vi "Using Connection Strings.vi"() -> ()   [LabVIEW 2012]
doc: "This example shows how to build an executable that uses the Database Connectivity Toolkit. It also shows how to dynamically create a connection string so the database being used can move with the executable."
uses:
  NI_Database_API_64.lvlib
  _DB Variant To Data/Database Variant To Data.xnode
  Connection.llb/DB Tools Open Connec (String).vi
  Auxilliary.llb/DB Tools Cursor Type.ctl
  Connection.llb/Conn Execute.vi
  Recordset.llb/Rec Get Recordset Properties (R).vi
  Recordset.llb/Rec Move To Record N (R).vi
  Recordset.llb/Rec Fetch Recordset Data (R).vi
  Recordset.llb/Rec Destroy - Connection.vi
panel:
  out "String read from database":string
  out "Numeric read from database":i32
  out "Date/Time read from database":timestamp format="%<%X\n%x>T"
  in  "String to insert":string="this is a test."
  in  "Numeric to insert":i32=125
  out "Date/Time inserted":timestamp format="%<%X\n%x>T"
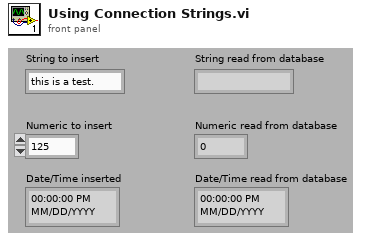
[diagram p1: front panel]
types:
  T1 = typedef "NI_Database_API_64.lvlib/DB Tools Cursor Type.ctl" = enum16{"forward-only", "keyset", "dynamic", "static"}
  T2 = enum32{"invalid app kind", "Development System", "Run Time System", "Student Edition", "Embedded LabVIEW", "Evaluation", "Custom"}
  T3 = typedef "NI_Database_API_64.lvlib/Conn ObjectReference.ctl" = refnum<k1>
  T4 = cluster{"String to insert":string, "Numeric to insert":i32, "seconds since 1Jan1904":timestamp}
  T5 = typedef "NI_Database_API_64.lvlib/Rec ObjectReference.ctl" = refnum<k1>
  T6 = typedef "NI_Database_API_64.lvlib/Rec Properties.ctl" = cluster{"column count":i32, "record index":i32, "record count":i32, "bof?":bool, "eof?":bool, "cursor type":T1, "cache size":i32, "state":enum16{"closed", "open"}}
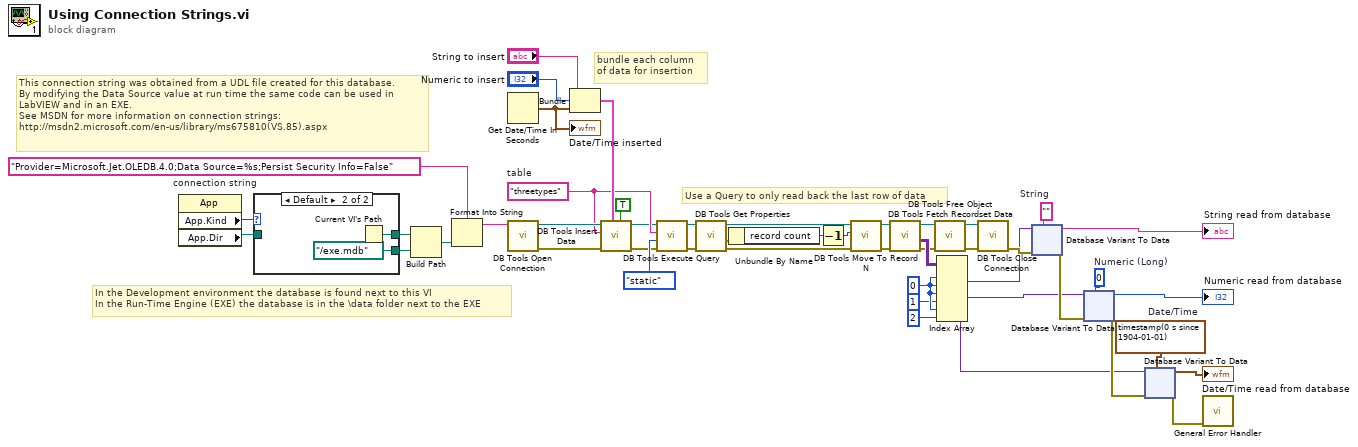
[diagram p0: block diagram]
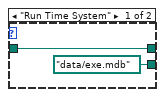
[diagram p2: hidden frame]
diagram:
  w3 = 0 ("disabled index (col)")
  w34 = timestamp(0 s since 1904-01-01)  # Date/Time
  w36 = "Provider=Microsoft.Jet.OLEDB.4.0;Data Source=%s;Persist Security Info=False"  # connection string
  w41 = 0  # Numeric (Long)
  w40 = ""  # String
  w10 = "threetypes"  # table
  # "This connection string was obtained from a UDL file created for this database.\nBy modifying the Data Source value at run time the same code can be used in\nLabVIEW and in an EXE.\nSee MSDN for more information on connection strings:\nhttp://msdn2.microsoft.com/en-us/library/ms675810(VS.85).aspx"
  # "In the Development environment the database is found next to this VI\nIn the Run-Time Engine (EXE) the database is in the \\data folder next to the EXE"
  # "Use a Query to only read back the last row of data"
  # "bundle each column\nof data for insertion"
  n1 = property class="App"() -> ("App.Kind"=w32:T2, "App.Dir"=w31:path)  [unwired: 2 in, 2 out]
  n2 = case shown="Default" w32 {
    tunnel: w31 -> [w50 _]
    tunnel: [path "data/exe.mdb" ("path") path "../exe.mdb" ("path")] -> w29
    tunnel: [w50 w51] -> w28
    frame "Run Time System" {
    }
    frame Default {
      n3 = Current VI's Path() -> (path=w51:path)
    }
  }
  n4 = Build Path(base path=w28, name or relative path=w29) -> (appended path=w30:path)
  n5 = Format Into String(format string=w36, w30) -> (resulting string=w35:string)  [unwired: 2 in, 1 out]
  n6 = Get Date/Time In Seconds() -> (seconds since 1Jan1904=w33:timestamp)
  "Date/Time inserted" <- w33
  n7 = call-poly "DB Tools Open Connection.vi"("connection information"=w35) -> ("error out"=w25:errorcluster, "connection reference"=w26:T3)  [unwired: 7 in]
  n8 = Bundle("String to insert"="String to insert", "Numeric to insert"="Numeric to insert", "seconds since 1Jan1904"=w33) -> (w48:T4)  [unwired: 1 in]
  n9 = call "DB Tools Insert Data.vi"("create table? (F)"=TRUE ("create table? (f)"), "data"=w48, "error in (no error)"=w25, "table"=w10, "connection reference"=w26) -> ("error out"=w7:errorcluster, "connection reference out"=w8:T3)  [unwired: 5 in]
  n10 = call-poly "DB Tools Execute Query.vi"("error in (no error)"=w7, "cursor type"=DB_Tools_Cursor_Type."static", "SQL query"=w10, "connection reference"=w8) -> ("error out"=w22:errorcluster, "recordset reference"=w23:T5)  [unwired: 4 in]
  n11 = call-poly "DB Tools Get Properties.vi"("error in (no error)"=w22, "recordset reference"=w23) -> ("error out"=w18:errorcluster, "recordset properties"=w21:T6, "recordset reference out"=w19:T5)  [unwired: 3 in]
  n12 = Unbundle By Name(w21) -> ("record count"=w20:i32)
  n13 = Decrement(x=w20) -> (x-1=w9:i32)
  n14 = call-poly "DB Tools Move To Record N.vi"("error in (no error)"=w18, "n (0)"=w9, "recordset reference"=w19) -> ("error out"=w17:errorcluster, "recordset reference out"=w16:T5)  [unwired: 7 in]
  n15 = call-poly "DB Tools Fetch Recordset Data.vi"("error in (no error)"=w17, "recordset reference"=w16) -> ("error out"=w12:errorcluster, "recordset data"=w15:variant[][], "recordset reference out"=w14:T5)  [unwired: 3 in]
  n16 = call-poly "DB Tools Free Object.vi"("error in (no error)"=w12, "recordset reference"=w14) -> ("error out"=w11:errorcluster, "connection reference"=w13:T3)  [unwired: 8 in]
  n17 = Index Array(array=w15, index (row) #1=w3, index (col) #1=w3, index (row) #2=w3, index (col) #2=1 ("disabled index (col)"), index (row) #3=w3, index (col) #3=2 ("disabled index (col)")) -> (element #1=w6:variant, element #2=w5:variant, element #3=w4:variant)
  n18 = call "DB Tools Close Connection.vi"("error in (no error)"=w11, "connection reference"=w13) -> ("error out"=w45:errorcluster)  [unwired: 5 in]
  n19 = xnode "Database Variant To Data"("database variant"=w6, "error in"=w45, "type"=w40) -> ("data"=→"String read from database":string, "error out"=w39:errorcluster)
  n20 = xnode "Database Variant To Data"("database variant"=w5, "error in"=w39, "type"=w41) -> ("data"=→"Numeric read from database":i32, "error out"=w37:errorcluster)
  n21 = xnode "Database Variant To Data"("database variant"=w4, "error in"=w37, "type"=w34) -> ("data"=→"Date/Time read from database":timestamp, "error out"=w38:errorcluster)
  n22 = call <vilib>:"General Error Handler.vi"("error in (no error)"=w38) -> ()  [unwired: 10 in, 5 out]
